vi "Set Name.vi"(8 "error in":errorcluster, 10 "Section Name":string, 11 "Object Entry in":refnum<class "Section.lvclass">) -> (0 "error out":errorcluster, 3 "Object Entry out":refnum<class "Section.lvclass">)   [LabVIEW 2019, in "Electronic Datasheet.lvlib" / "Section.lvclass"]
uses:
  Section.lvclass
  Section.lvclass/Section.ctl
  Section Name/Section Name.lvclass
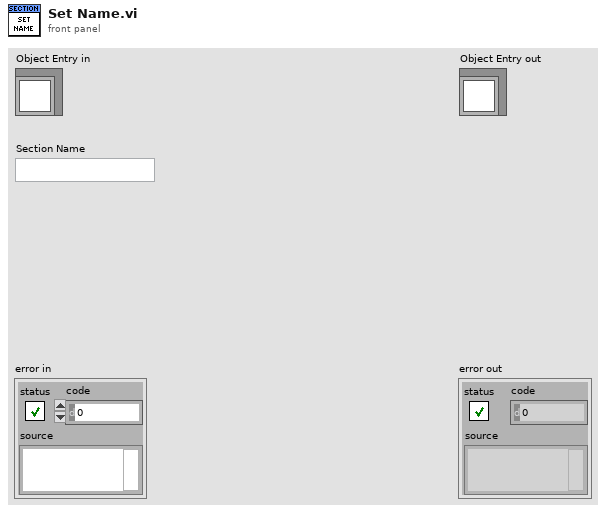
[diagram p1: front panel]
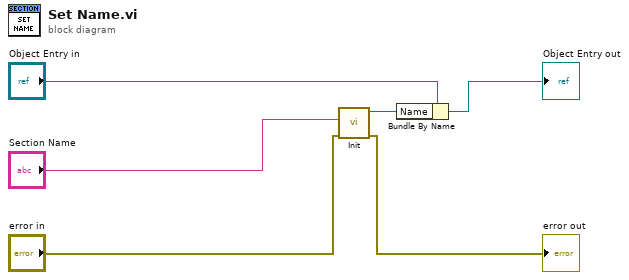
[diagram p0: block diagram]
diagram:
  n1 = call "Init.vi"("error in"="error in", "Section Name"="Section Name") -> ("error out"=→"error out":errorcluster, "Section Name out"=w3:refnum<class "Section Name.lvclass">)  [unwired: 8 in]
  n2 = Bundle By Name(cluster="Object Entry in", "Name"=w3) -> (→"Object Entry out":refnum<class "Section.lvclass">)
